vi "TotalScanTime (SubVI).vi"(9 "TblParam":sgl[][](array[numeric]), 11 "NTick":i32) -> (3 "sum":dbl)   [LabVIEW 2017]
panel:
  out "Array":dbl[](array[numeric])
  out "Numeric":i32
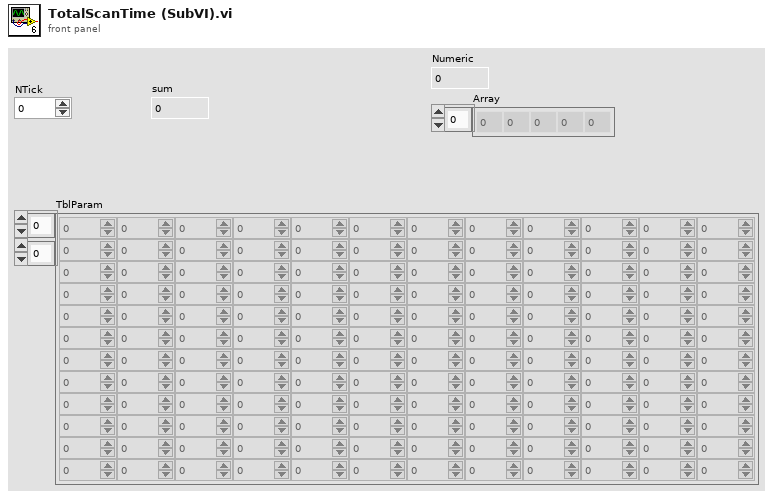
[diagram p1: front panel]
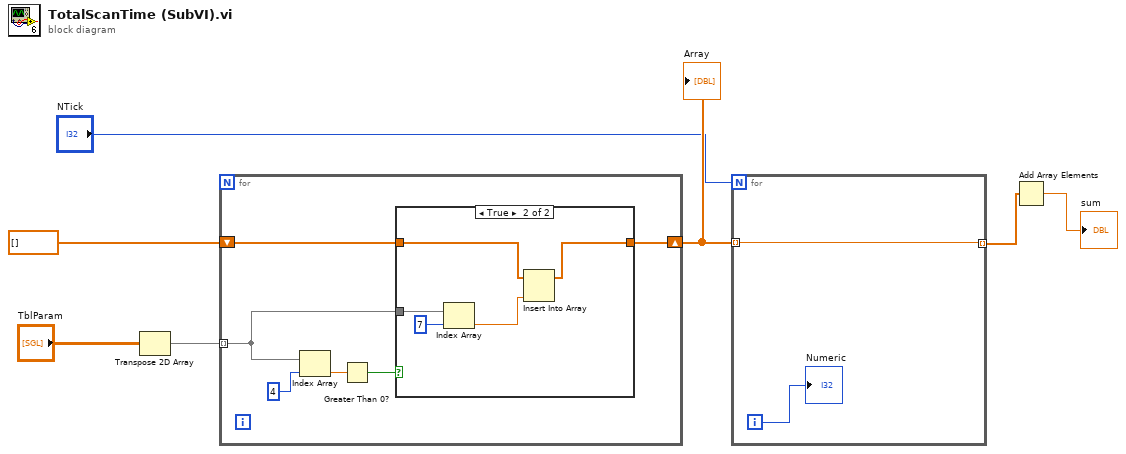
[diagram p0: block diagram]
diagram:
  n1 = Transpose 2D Array(2D array="TblParam") -> (transposed array=w3:sgl[][])
  n2 = for {
    tunnel: w3 -> [w10] mode=indexing
    shift-right: [w8] -> w7
    shift-left: dbl[] [] ("Array") -> [w9]
    n3 = Index Array(array=w10, index=4) -> (element=w12:sgl)
    n4 = Greater Than 0?(x=w12) -> (x > 0?=w11:bool)
    n5 = case shown="True" w11 {
      tunnel: w10 -> [_ w19]
      tunnel: w9 -> [w14 w16]
      tunnel: [w14 w15] -> w8
      frame False {
      }
      frame True {
        n6 = Index Array(array=w19, index=7) -> (element=w17:sgl)
        n7 = Insert Into Array(array=w16, new element=w17) -> (w15:dbl[])  [unwired: 1 in]
      }
    }
  }
  "Array" <- w7
  n8 = for {
    N: "NTick" -> [_]
    tunnel: w7 -> [w21] mode=indexing
    tunnel: [w21] -> w2 mode=indexing
    i -> [w20]
    "Numeric" <- w20
  }
  n9 = Add Array Elements(numeric array=w2) -> (sum=→"sum":dbl)
